vi "Delete Cluster Controls.vi"(8 "error in (no error)":errorcluster, 11 "Cluster in":refnum<vi>) -> (0 "error out":errorcluster, 3 "Cluster out":refnum<vi>)   [LabVIEW 2019, in "gRPC Scripting Tools.lvlib"]
uses:
  gRPC Scripting Tools.lvlib
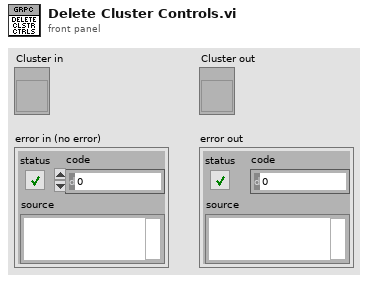
[diagram p1: front panel]
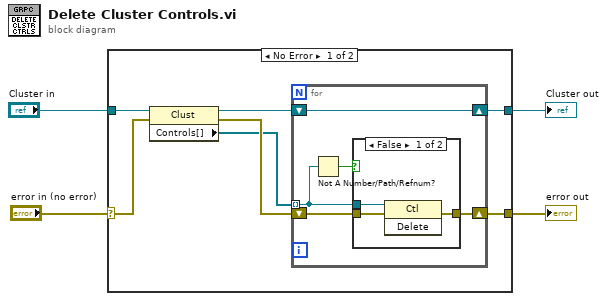
[diagram p0: block diagram]
diagram:
  n1 = case shown="No Error" "error in (no error)" {
    selector: "error in (no error)" -> [w10 w22]
    tunnel: [w5 w21] -> w4
    tunnel: "Cluster in" -> [w11 w21]
    tunnel: [w7 w22] -> w1
    frame No Error {
      n2 = property class="Clust"(reference=w11, error in=w10) -> (reference out=w6:refnum<vi>, error out=w9:errorcluster, "Controls[]"=w8:refnum<vi>[])
      n3 = for {
        tunnel: w8 -> [w12] mode=indexing
        shift-right: [w16] -> w7
        shift-left: w9 -> [w13]
        shift-right: [w15] -> w5
        shift-left: w6 -> [w15]
        n4 = Not A Number/Path/Refnum?(number/path/refnum=w12) -> (NaN/Path/Refnum?=w14:bool)
        n5 = case shown="False" w14 {
          tunnel: [w19 w20] -> w16
          tunnel: w13 -> [w18 w20]
          tunnel: w12 -> [w17 _]
          frame False {
            n6 = invoke class="Ctl" method="Delete"(reference=w17, error in=w18) -> (error out=w19:errorcluster)  [unwired: 1 in, 2 out]
          }
          frame True {
          }
        }
      }
    }
    frame Error {
    }
  }
  "Cluster out" <- w4
  "error out" <- w1
